vi "Intake Control Loop.vi"() -> ()   [LabVIEW 2018]
uses:
  <vilib>/Rock Robotics/WPI/ThirdParty/Phoenix-LabVIEW/Motor Controller/Controls/CTRE_Phoenix_MotorControl_NeutralMode.ctl
  <vilib>/Rock Robotics/WPI/ThirdParty/Phoenix-LabVIEW/Motor Controller/Controls/CTRE_Phoenix_MotorControl_ControlMode.ctl
  Infrastructure/RobotMap.vi
  Robot Global Data.vi
  <vilib>/Rock Robotics/WPI/ThirdParty/Phoenix-LabVIEW/Motor Controller/Get/CTRE_Phoenix_MotorController_GetOutputCurrent_Enhanced.vi
  <vilib>/Rock Robotics/Network Tables/NT Read Boolean.vi
  <vilib>/Rock Robotics/WPI/ThirdParty/Phoenix-LabVIEW/Motor Controller/Get/CTRE_Phoenix_MotorController_GetSelectedSensorData.vi
  <vilib>/Rock Robotics/Network Tables/NT Write Number.vi
panel:
  in  "Cargo Current Threshold when the ball is in intake":dbl=5.0
  out "Hatch Velocity":i32(graph)
  out "Hatch Position":i32(graph)
  # "Not an actual number atm"
  # "Cargo Positive Must Be IN"
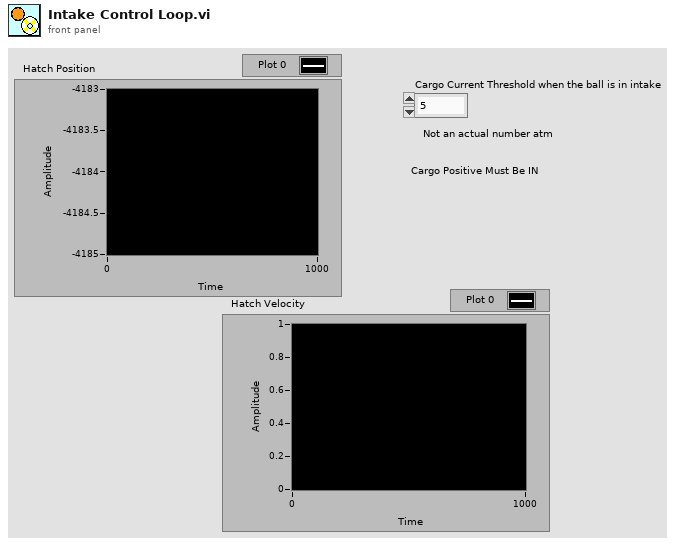
[diagram p1: front panel]
types:
  T1 = enum16{"FollowerType_PercentOutput", "FollowerType_AuxOutput1"}
  T2 = typedef "CTRE_Phoenix_MotorControl_NeutralMode.ctl" = enum8{"EEPROMSetting", "Override to Coast", "Override to Brake"}
  T3 = typedef "WPI_MotorControlDeviceRef.ctl" = cluster{"DeviceStatus":errorcluster, "Type":T4, "PWM":cluster{"PWM Channel":T5, "DeadBand":T6}, "CAN":cluster{"Device Number":u8, "SetOutput VI Ref":variant, "GetOutput VI Ref":variant, "Enable VI Ref":variant, "Disable VI Ref":variant, "Data":variant}, "Invert":bool, "DIO PWM":cluster{"PWM \"Enable\" Channel":T5, "DIOChannel":T7, "PWM Rate":dbl}}
  T4 = typedef "WPI_MotorControlType.ctl" = enum16{"PWM", "CAN", "DIO PWM"}
  T5 = typedef "FPGA_DIOPWMChannel.ctl" = enum8{"PWM 0", "PWM 1", "PWM 2", "PWM 3", "PWM 4", "PWM 5", "PWM 6", "PWM 7", "PWM 8", "PWM 9", "PWM MXP 0", "PWM MXP 1", "PWM MXP 2", "PWM MXP 3", "PWM MXP 4", "PWM MXP 5", "PWM MXP 6", "PWM MXP 7", "PWM MXP 8", "PWM MXP 9", "Invalid"}
  T6 = typedef "WPI_PWMDeadband.ctl" = cluster{"Name":string, "maxPositivePwm":i32, "minPositivePwm":i32, "centerPwm":i32, "maxNegativePwm":i32, "minNegativePwm":i32, "angularRange":u16}
  T7 = typedef "FPGA_DIOChannel.ctl" = enum8{"DIO 0", "DIO 1", "DIO 2", "DIO 3", "DIO 4", "DIO 5", "DIO 6", "DIO 7", "DIO 8", "DIO 9", "DIO MXP 0", "DIO MXP 1", "DIO MXP 2", "DIO MXP 3", "DIO MXP 4", "DIO MXP 5", "DIO MXP 6", "DIO MXP 7", "DIO MXP 8", "DIO MXP 9", "DIO MXP 10", "DIO MXP 11", "DIO MXP 12", "DIO MXP 13", "DIO MXP 14", "DIO MXP 15", "SPI Port CS1", "SPI Port CS2", "SPI Port CS3", "SPI Port MISO", "SPI Port MOSI", "Invalid"}
  T8 = typedef "CTRE_Phoenix_MotorControl_ControlMode.ctl" = u16
  T9 = cluster{"Position (Raw Sensor Units)":i32, "Velocity (Raw Sensor Units per 100 ms)":i32}
  T10 = cluster{"Cargo Motor Value":dbl, "Hatch Setpoint":dbl}
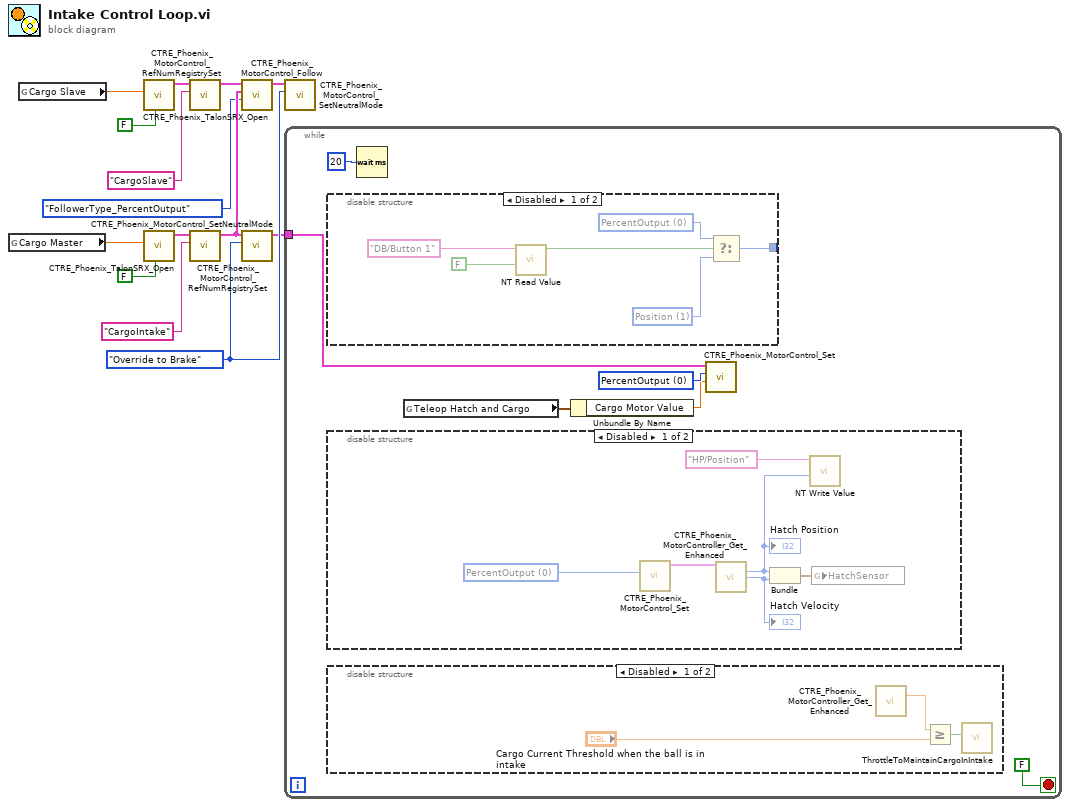
[diagram p0: block diagram]
diagram:
  w8 = CTRE_Phoenix_MotorControl_NeutralMode."Override to Brake" ("Motor Control Neutral Mode")
  n1 = global read "RobotMap.vi" "Cargo Master"() -> (w12:dbl)
  n2 = global read "RobotMap.vi" "Cargo Slave"() -> (w11:dbl)
  n3 = call <vilib>:"CTRE_Phoenix_TalonSRX_Open.vi"("Invert"=FALSE, "Device Number"=w11) -> ("CAN Talon SRX Ref"=w13:T3)  [unwired: 8 in, 1 out]
  n4 = call <vilib>:"CTRE_Phoenix_TalonSRX_Open.vi"("Invert"=FALSE, "Device Number"=w12) -> ("CAN Talon SRX Ref"=w14:T3)  [unwired: 8 in, 1 out]
  n5 = call <vilib>:"CTRE_Phoenix_MotorControl_RefNumRegistrySet.vi"("refnum name"="CargoSlave", "PhoenixMotorControlDevRef"=w13) -> ("PhoenixMotorControlDevRef"=w5:T3)  [unwired: 8 in, 1 out]
  n6 = call <vilib>:"CTRE_Phoenix_MotorControl_RefNumRegistrySet.vi"("refnum name"="CargoIntake", "PhoenixMotorControlDevRef"=w14) -> ("PhoenixMotorControlDevRef"=w4:T3)  [unwired: 8 in, 1 out]
  n7 = call <vilib>:"CTRE_Phoenix_MotorControl_Follow.vi"("FollowerType"=T1."FollowerType_PercentOutput", "Master Controller to Follow"=w4, "PhoenixMotorControlDevRef"=w5) -> ("PhoenixMotorControlDevRef"=w1:T3)  [unwired: 7 in, 1 out]
  n8 = call <vilib>:"CTRE_Phoenix_MotorControl_SetNeutralMode.vi"("Motor Control Neutral Mode"=w8, "PhoenixMotorControlDevRef"=w4) -> ("PhoenixMotorControlDevRef"=w7:T3)  [unwired: 8 in, 1 out]
  n9 = call <vilib>:"CTRE_Phoenix_MotorControl_SetNeutralMode.vi"("Motor Control Neutral Mode"=w8, "PhoenixMotorControlDevRef"=w1) -> ()  [unwired: 8 in, 2 out]
  n10 = while {
    tunnel: w7 -> [w15]
    stop <- FALSE stop-if-true
    w20 = T8 0 items=["PercentOutput"=0, "Position"=1, "Velocity"=2, "Current"=3, "Follower"=5, "MotionProfile"=6, "MotionMagic"=7, "MotionProfileArc"=10, "Disabled"=15] ("Control Mode")
    n11 = disable-structure shown="Disabled" {
      disable-tunnel: [w31 _] -> _
      frame Disabled {
        w29 = T8 1 items=["PercentOutput"=0, "Position"=1, "Velocity"=2, "Current"=3, "Follower"=5, "MotionProfile"=6, "MotionMagic"=7, "MotionProfileArc"=10, "Disabled"=15] ("Control Mode")
        w30 = T8 0 items=["PercentOutput"=0, "Position"=1, "Velocity"=2, "Current"=3, "Follower"=5, "MotionProfile"=6, "MotionMagic"=7, "MotionProfileArc"=10, "Disabled"=15] ("Control Mode")
        n12 = call-poly <vilib>:"NT Read Value.vi"("Default Value"=FALSE, "Name"="DB/Button 1") -> ("Boolean"=w28:bool)  [unwired: 8 in, 1 out]
        n13 = Select(t=w30, s=w28, f=w29) -> (s? t:f=w31:T8)
      }
      frame Enabled {
      }
    }
    n14 = disable-structure shown="Disabled" {
      frame Disabled {
        w21 = T8 0 items=["PercentOutput"=0, "Position"=1, "Velocity"=2, "Current"=3, "Follower"=5, "MotionProfile"=6, "MotionMagic"=7, "MotionProfileArc"=10, "Disabled"=15] ("Control Mode")
        n15 = call <vilib>:"CTRE_Phoenix_MotorControl_Set.vi"("Control Mode"=w21) -> ("PhoenixMotorControlDevRef"=w26:T3)  [unwired: 9 in, 1 out]
        n16 = call-poly <vilib>:"CTRE_Phoenix_MotorController_Get_Enhanced.vi"("PhoenixMotorControlDevRef"=w26) -> ("Position (Raw Sensor Units)"=w22:i32, "Velocity (Raw Sensor Units per 100 ms)"=w24:i32)  [unwired: 11 in, 2 out]
        "Hatch Position" <- w22
        "Hatch Velocity" <- w24
        n17 = Bundle("Position (Raw Sensor Units)"=w22, "Velocity (Raw Sensor Units per 100 ms)"=w24) -> (w25:T9)  [unwired: 1 in]
        n18 = call-poly <vilib>:"NT Write Value.vi"("Numeric"=w22, "Name"="HP/Position") -> ()  [unwired: 9 in, 1 out]
        n19 = global write "Robot Global Data.vi" "HatchSensor"(w25) -> ()
      }
      frame Enabled {
      }
    }
    n20 = disable-structure shown="Disabled" {
      frame Disabled {
        n21 = call-poly <vilib>:"CTRE_Phoenix_MotorController_Get_Enhanced.vi"() -> ("Output Current"=w35:dbl)  [unwired: 13 in, 2 out]
        n22 = Greater Or Equal?(x=w35, y="Cargo Current Threshold when the ball is in intake") -> (x >= y?=w33:bool)
        n23 = call "ThrottleToMaintainCargoInIntake.vi"("Current above threshold?"=w33) -> ()  [unwired: 10 in, 1 out]
      }
      frame Enabled {
      }
    }
    n24 = Wait (ms)(milliseconds to wait=u32 20) -> ()  [unwired: 1 out]
    n25 = global read "Robot Global Data.vi" "Teleop Hatch and Cargo"() -> (w17:T10)
    n26 = Unbundle By Name(w17) -> ("Cargo Motor Value"=w16:dbl)
    n27 = call <vilib>:"CTRE_Phoenix_MotorControl_Set.vi"("Output"=w16, "Control Mode"=w20, "PhoenixMotorControlDevRef"=w15) -> ()  [unwired: 7 in, 2 out]
  }
